vi "抽奖机.vi"() -> ()   [LabVIEW 2018]
panel:
  out "字符串":string
  out "日期/时间字符串":string
  out "数值 5":dbl
  out "数值 4":dbl
  out "数值 3":dbl
  out "数值 2":dbl
  out "数值":dbl
  out "led10":bool
  out "led9":bool
  out "led8":bool
  out "led7":bool
  out "led6":bool
  out "led5":bool
  out "led4":bool
  out "led3":bool
  out "led2":bool
  out "led11 2":bool
  in  "停止/抽奖":bool
  out "led11":bool
  out "led17":bool
  out "led18":bool
  out "led16":bool
  out "led15":bool
  out "led12":bool
  out "led13":bool
  out "led14":bool
  out "led20":bool
  out "led19":bool
  in  "关机":bool
  out "期数":dbl
  # "第"
  # "期"
  # "抽奖"
  # "停止"
  # "中奖时间"
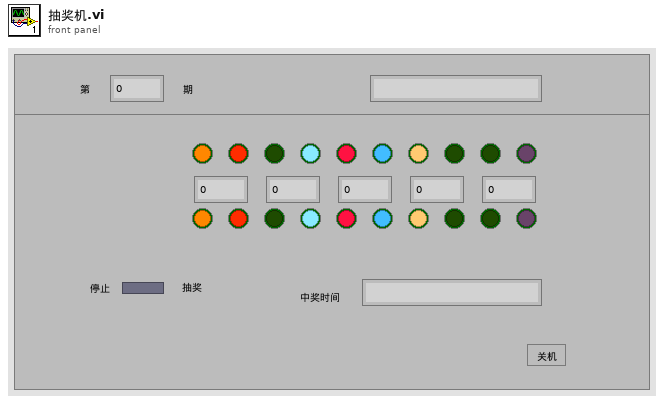
[diagram p1: front panel]
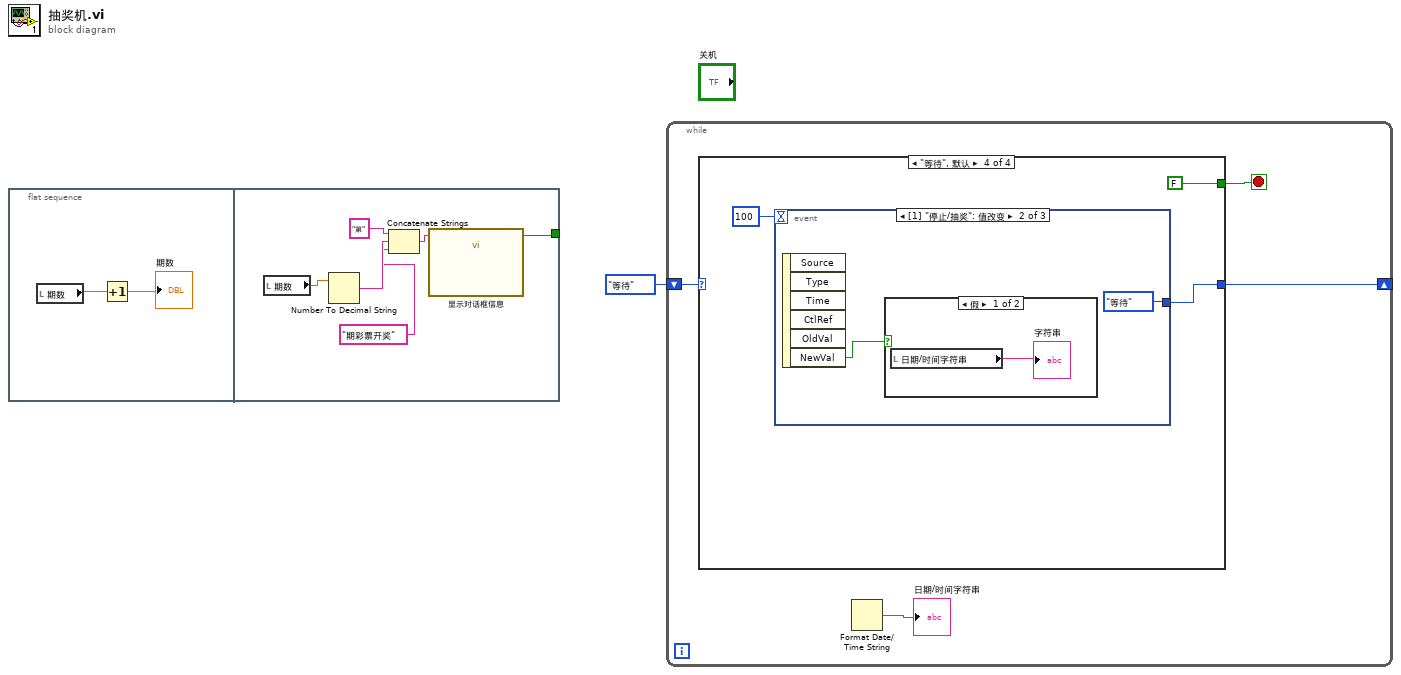
[diagram p0: block diagram]
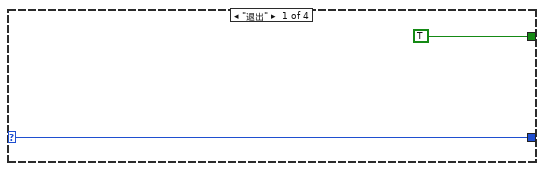
[diagram p2: hidden frame]
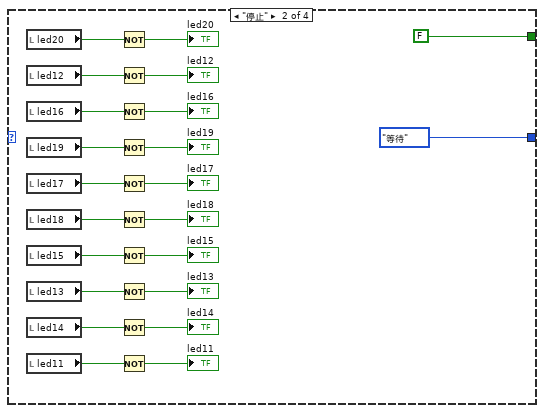
[diagram p3: hidden frame]
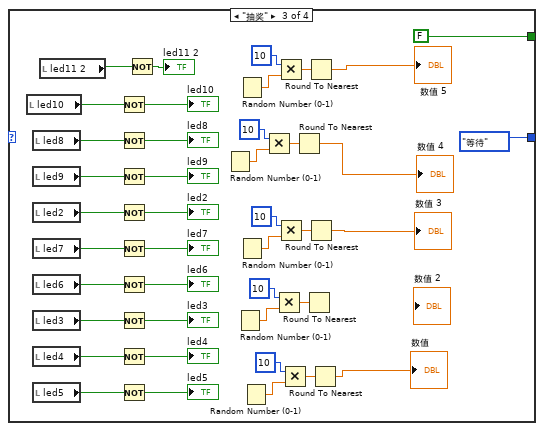
[diagram p4: hidden frame]
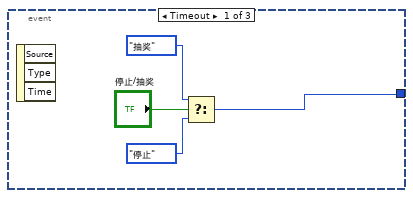
[diagram p5: hidden frame]
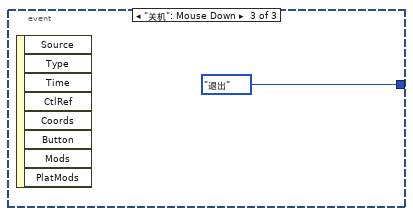
[diagram p7: hidden frame]
diagram:
  n1 = flat-sequence {
    tunnel: [w4] -> _
    frame #0 {
      n2 = local read "期数"() -> (w3:dbl)
      n3 = Increment(x=w3) -> (x+1=→"期数":dbl)
    }
    frame #1 {
      n4 = local read "期数"() -> (w8:dbl)
      n5 = Number To Decimal String(number=w8) -> (decimal integer string=w7:string)  [unwired: 1 in]
      n6 = Concatenate Strings("第", w7, "期彩票开奖") -> (w5:string)
      n7 = call "显示对话框信息"("Message"=w5) -> ("确定"=w4:bool)  [unwired: 9 in, 1 out]
    }
  }
  n8 = while {
    shift-right: [w11] -> _
    shift-left: enum16{"退出", "停止", "抽奖", "等待"}."等待" -> [w13]
    stop <- w12 stop-if-true
    n9 = case shown="\"等待\", 默认" w13 {
      selector: w13 -> [w14 _ _ _]
      tunnel: [TRUE FALSE FALSE FALSE] -> w12
      tunnel: [w14 enum16{"退出", "停止", "抽奖", "等待"}."等待" enum16{"退出", "停止", "抽奖", "等待"}."等待" w80] -> w11
      frame "退出" {
      }
      frame "停止" {
        n10 = local read "led20"() -> (w18:bool)
        n11 = local read "led12"() -> (w19:bool)
        n12 = local read "led16"() -> (w22:bool)
        n13 = local read "led19"() -> (w23:bool)
        n14 = local read "led17"() -> (w26:bool)
        n15 = local read "led18"() -> (w27:bool)
        n16 = local read "led15"() -> (w30:bool)
        n17 = local read "led13"() -> (w31:bool)
        n18 = local read "led14"() -> (w34:bool)
        n19 = local read "led11"() -> (w35:bool)
        n20 = Not(x=w18) -> (.not. x?=→"led20":bool)
        n21 = Not(x=w19) -> (.not. x?=→"led12":bool)
        n22 = Not(x=w22) -> (.not. x?=→"led16":bool)
        n23 = Not(x=w23) -> (.not. x?=→"led19":bool)
        n24 = Not(x=w26) -> (.not. x?=→"led17":bool)
        n25 = Not(x=w27) -> (.not. x?=→"led18":bool)
        n26 = Not(x=w30) -> (.not. x?=→"led15":bool)
        n27 = Not(x=w31) -> (.not. x?=→"led13":bool)
        n28 = Not(x=w34) -> (.not. x?=→"led14":bool)
        n29 = Not(x=w35) -> (.not. x?=→"led11":bool)
      }
      frame "抽奖" {
        n30 = local read "led10"() -> (w60:bool)
        n31 = local read "led8"() -> (w61:bool)
        n32 = local read "led9"() -> (w64:bool)
        n33 = local read "led2"() -> (w65:bool)
        n34 = local read "led7"() -> (w68:bool)
        n35 = local read "led6"() -> (w69:bool)
        n36 = local read "led3"() -> (w72:bool)
        n37 = local read "led4"() -> (w73:bool)
        n38 = local read "led5"() -> (w76:bool)
        n39 = local read "led11 2"() -> (w57:bool)
        n40 = Not(x=w60) -> (.not. x?=→"led10":bool)
        n41 = Not(x=w61) -> (.not. x?=→"led8":bool)
        n42 = Not(x=w64) -> (.not. x?=→"led9":bool)
        n43 = Not(x=w65) -> (.not. x?=→"led2":bool)
        n44 = Not(x=w68) -> (.not. x?=→"led7":bool)
        n45 = Not(x=w69) -> (.not. x?=→"led6":bool)
        n46 = Not(x=w72) -> (.not. x?=→"led3":bool)
        n47 = Not(x=w73) -> (.not. x?=→"led4":bool)
        n48 = Not(x=w76) -> (.not. x?=→"led5":bool)
        n49 = Not(x=w57) -> (.not. x?=→"led11 2":bool)
        n50 = Random Number (0-1)() -> (number: 0 to 1=w46:dbl)
        n51 = Random Number (0-1)() -> (number: 0 to 1=w52:dbl)
        n52 = Random Number (0-1)() -> (number: 0 to 1=w43:dbl)
        n53 = Random Number (0-1)() -> (number: 0 to 1=w49:dbl)
        n54 = Random Number (0-1)() -> (number: 0 to 1=w56:dbl)
        n55 = Multiply(x=10, y=w46) -> (x*y=w44:dbl)
        n56 = Multiply(x=10, y=w52) -> (x*y=w50:dbl)
        n57 = Multiply(x=10, y=w43) -> (x*y=w41:dbl)
        n58 = Multiply(x=10, y=w49) -> (x*y=w47:dbl)
        n59 = Multiply(x=10, y=w56) -> (x*y=w54:dbl)
        n60 = Round To Nearest(number=w44) -> (nearest integer value=→"数值 4":dbl)
        n61 = Round To Nearest(number=w50) -> ()  [unwired: 1 out]
        n62 = Round To Nearest(number=w41) -> (nearest integer value=→"数值 5":dbl)
        n63 = Round To Nearest(number=w47) -> (nearest integer value=→"数值 3":dbl)
        n64 = Round To Nearest(number=w54) -> (nearest integer value=→"数值":dbl)
      }
      frame "等待", Default {
        n65 = event shown="[1] \"停止/抽奖\": 值改变" {
          selector: _ -> [_ _ _]
          dyn-events: _ -> [_ _ _]
          timeout: 100 -> [_ _ _]
          tunnel: [w82 enum16{"退出", "停止", "抽奖", "等待"}."等待" enum16{"退出", "停止", "抽奖", "等待"}."退出"] -> w80
          event Timeout {
            n66 = event-data() -> ()  [unwired: 1 in, 3 out]
            n67 = Select(t=enum16{"退出", "停止", "抽奖", "等待"}."抽奖", s="停止/抽奖", f=enum16{"退出", "停止", "抽奖", "等待"}."停止") -> (s? t:f=w82:enum16{"退出", "停止", "抽奖", "等待"})
          }
          event "停止/抽奖": Value Change {
            n68 = event-data() -> ("NewVal"=w87:bool)  [unwired: 1 in, 5 out]
            n69 = case shown="假" w87 {
              frame False {
                n70 = local read "日期/时间字符串"() -> (→"字符串":string)
              }
              frame True {
              }
            }
          }
          event "关机": Mouse Down {
            n71 = event-data() -> ()  [unwired: 1 in, 8 out]
          }
        }
      }
    }
    n72 = Format Date/Time String() -> (date/time string=→"日期/时间字符串":string)  [unwired: 3 in]
  }
